vi "Launcher.vi"() -> ()   [LabVIEW 2020]
uses:
  UI Actor.lvclass
  C:/Program Files/National Instruments/LabVIEW 2020/vi.lib/ActorFramework/Actor/Actor.lvclass
  UI Actor.lvclass/UI Actor.ctl
  Write Productos.vi
  Write Monedas.vi
  <vilib>/ActorFramework/Actor/Actor.lvclass
panel:
  in  "Monedas":enum16{"USD", "MXN"}(ring)
  in  "Productos":enum16{"Nestle", "Coca"}(ring)
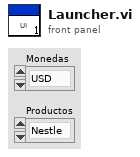
[diagram p1: front panel]
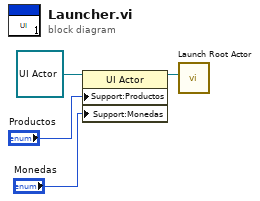
[diagram p0: block diagram]
diagram:
  n1 = property class="UI Actor"(reference=refnum<class "UI Actor.lvclass"> refnum ("UI Actor.lvlib:UI Actor.lvclass"), "Support:Productos"="Productos", "Support:Monedas"="Monedas") -> (reference out=w3:refnum<class "UI Actor.lvclass">)  [unwired: 1 in, 1 out]
  n2 = call <vilib>:"Launch Root Actor.vi"("Actor"=w3) -> ()  [unwired: 9 in, 2 out]
